vi "10-100.vi"() -> ()   [LabVIEW 2015]
uses:
  <vilib>/NXT/Block Support/NXT_InputPort.ctl
  <vilib>/NXT/Block Support/NXT_OutputPort.ctl
  <vilib>/NXT/Dual Mode Library/Sensors/Sonar_cm.vi
  <vilib>/NXT/NXTIO Xnodes/NXTIONodeSubVIs/NXTMoveMotors.vi
  <vilib>/NXT/Dual Mode Library/Sensors/Light_On.vi
  <vilib>/NXT/NXTIO Xnodes/NXTIONodeSubVIs/LEGOStopAllMotors.vi
  <vilib>/NXT/Dual Mode Library/Waits/Wait_Num.vi
  <vilib>/NXT/Dual Mode Library/Sensors/Touch_Pressed.vi
  <vilib>/NXT/Subs/LVHSConnector.ctl
  <vilib>/NXT/NXTIO Xnodes/AddressXNode/NXTIOAddress.xnode
  <vilib>/NXT/NXTIO Xnodes/NXTIOXNode/NXTIO.xnode
  <vilib>/NXT/LegoClasses/BrickReference/BrickReference.lvclass
panel:
  in  "stop":bool
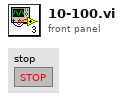
[diagram p1: front panel]
types:
  T1 = typedef "NXT_OutputPort.ctl" = u8
  T2 = typedef "NXT_InputPort.ctl" = u32
  T3 = typedef "LVHSConnector.ctl" = refnum<class "BrickReference.lvclass">
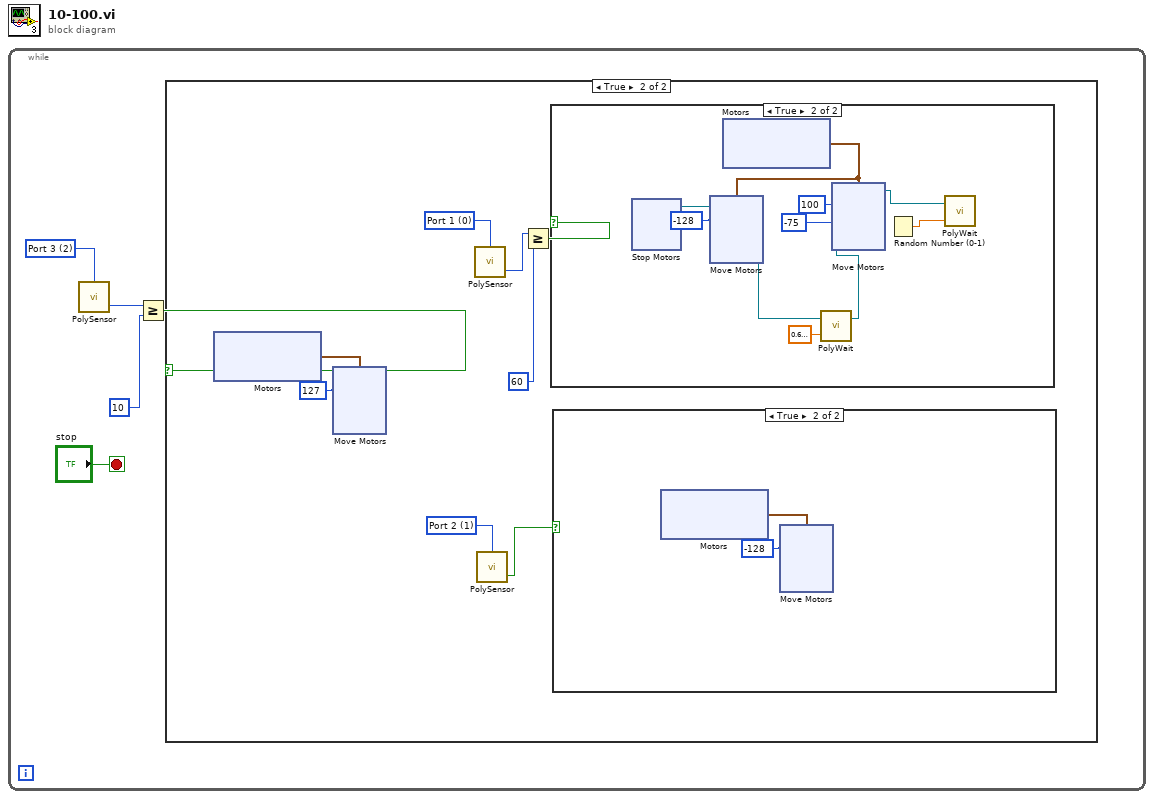
[diagram p0: block diagram]
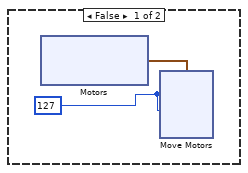
[diagram p2: hidden frame]
diagram:
  n1 = while {
    stop <- "stop" stop-if-true
    w5 = T2 2 items=["Port 1", "Port 2", "Port 3", "Port 4"] ("Port (Port 4)")
    n2 = call-poly <vilib>:"PolySensor.vi"("Port (Port 4)"=w5) -> ("Distance (cm)"=w4:i16)  [unwired: 2 in, 1 out]
    n3 = Greater Or Equal?(x=w4, y=i16 10) -> (x >= y?=w2:bool)
    n4 = case shown="True" w2 {
      frame False {
        w6 = i8 127 ("Power/Speed 1")
        n5 = xnode "Motors"() -> ("Motor"=w7:cluster{"Port":T1, "Port":T1})
        n6 = xnode "Move Motors"("Power/Speed 2"=w6, "Power/Speed 1"=w6, "Motors"=w7) -> ()  [unwired: 1 in, 1 out]
      }
      frame True {
        w18 = T2 1 items=["Port 1", "Port 2", "Port 3", "Port 4"] ("Port (Port 3)")
        w19 = i8 127 ("Power/Speed 1")
        w21 = T2 0 items=["Port 1", "Port 2", "Port 3", "Port 4"] ("Port (Port 3)")
        n7 = xnode "Motors"() -> ("Motor"=w20:cluster{"Port":T1, "Port":T1})
        n8 = xnode "Move Motors"("Power/Speed 1"=w19, "Motors"=w20, "Power/Speed 2"=w19) -> ()  [unwired: 1 in, 1 out]
        n9 = call-poly <vilib>:"PolySensor.vi"("Port (Port 3)"=w21) -> ("Scaled Value"=w23:i16)  [unwired: 2 in, 1 out]
        n10 = call-poly <vilib>:"PolySensor.vi"("Port (Port 1)"=w18) -> ("Yes / No"=w17:bool)  [unwired: 2 in, 1 out]
        n11 = Greater Or Equal?(x=w23, y=i16 60) -> (x >= y?=w24:bool)
        n12 = case shown="True" w24 {
          frame False {
          }
          frame True {
            w50 = i8 -128 ("Power/Speed 1")
            n13 = xnode "Stop Motors"() -> ("NXT/EV3"=w46:T3)  [unwired: 2 in]
            n14 = xnode "Motors"() -> ("Motor"=w51:cluster{"Port":T1, "Port":T1})
            n15 = xnode "Move Motors"("Power/Speed 2"=w50, "Power/Speed 1"=w50, "Motors"=w51, "NXT/EV3"=w46) -> ("NXT/EV3"=w49:T3)
            n16 = call-poly <vilib>:"PolyWait.vi"("Time (1 sec)"=sgl 0.7, "NXT/EV3"=w49) -> ("NXT/EV3"=w48:T3)  [unwired: 2 in]
            n17 = xnode "Move Motors"("Power/Speed 2"=i8 -75, "Power/Speed 1"=i8 100, "Motors"=w51, "NXT/EV3"=w48) -> ("NXT/EV3"=w54:T3)
            n18 = Random Number (0-1)() -> (number: 0 to 1=w45:dbl)
            n19 = call-poly <vilib>:"PolyWait.vi"("Time (1 sec)"=w45, "NXT/EV3"=w54) -> ()  [unwired: 2 in, 1 out]
          }
        }
        n20 = case shown="True" w17 {
          frame False {
          }
          frame True {
            w25 = i8 -128 ("Power/Speed 1")
            n21 = xnode "Motors"() -> ("Motor"=w26:cluster{"Port":T1, "Port":T1})
            n22 = xnode "Move Motors"("Power/Speed 1"=w25, "Motors"=w26, "Power/Speed 2"=w25) -> ()  [unwired: 1 in, 1 out]
          }
        }
      }
    }
  }
